vi "Setup.vi"(8 "Error In":errorcluster, 10 "Data":refnum<class "Datum.lvclass">, 11 "Value":string) -> (0 "Error Out":errorcluster, 2 "Abstract Syntax Tree":refnum<class "Root.lvclass">, 3 "Renderer":refnum<class "Renderer.lvclass">)   [LabVIEW 2018, in "Tests.lvlib" / "Render.lvlib"]
uses:
  Render.lvlib
  src/Toolkit/Low-Level/Nodes/Root/Root.lvclass
  src/Toolkit/Low-Level/Renderer/Renderer.lvclass
  src/Toolkit/Data/Datum/Datum.lvclass
  src/Toolkit/Low-Level/Writers/String/String.lvclass
  D:/Users/cfield/Code/Field R&D Services/Labstache/src/Toolkit/Low-Level/Writers/Writer/Writer.lvclass
  src/Toolkit/Low-Level/Readers/String/String.lvclass
  D:/Users/cfield/Code/Field R&D Services/Labstache/src/Toolkit/Low-Level/Readers/Reader/Reader.lvclass
  src/Toolkit/Low-Level/Lexer/Lexer.lvclass
  src/Toolkit/Low-Level/Parser/Parser.lvclass
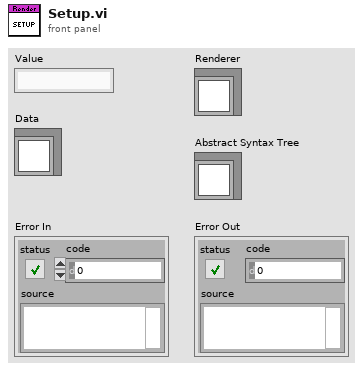
[diagram p1: front panel]
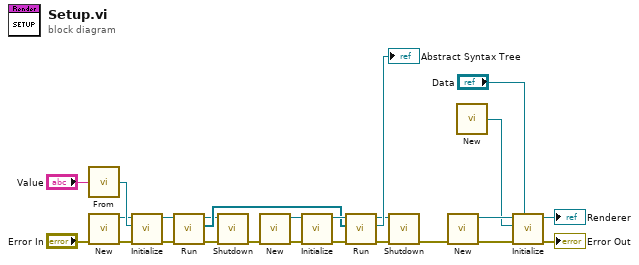
[diagram p0: block diagram]
diagram:
  n1 = call "From.vi"("Value"="Value") -> ("String"=w3:refnum<class "String.lvclass">)
  n2 = call "New.vi"("Error In"="Error In") -> ("Error Out"=w1:errorcluster, "Lexer"=w2:refnum<class "Lexer.lvclass">)  [unwired: 9 in]
  n3 = call-dynamic "Initialize.vi"("Error In"=w1, "Reader"=w3, "Lexer In"=w2) -> ("Error Out"=w11:errorcluster, "Lexer Out"=w10:refnum<class "Lexer.lvclass">)  [unwired: 7 in]
  n4 = call-dynamic "Run.vi"("Error In"=w11, "Lexer In"=w10) -> ("Error Out"=w12:errorcluster, "Tokens"=w14:refnum<class "Token.lvclass">[], "Lexer Out"=w13:refnum<class "Lexer.lvclass">)  [unwired: 7 in]
  n5 = call-dynamic "Shutdown.vi"("Error In"=w12, "Lexer In"=w13) -> ("Error Out"=w19:errorcluster)  [unwired: 7 in, 2 out]
  n6 = call "New.vi"("Error In"=w19) -> ("Error Out"=w20:errorcluster, "Parser"=w21:refnum<class "Parser.lvclass">)  [unwired: 9 in]
  n7 = call-dynamic "Initialize.vi"("Error In"=w20, "Parser In"=w21) -> ("Error Out"=w16:errorcluster, "Parser Out"=w15:refnum<class "Parser.lvclass">)  [unwired: 8 in]
  n8 = call-dynamic "Run.vi"("Error In"=w16, "Tokens"=w14, "Parser In"=w15) -> ("Error Out"=w17:errorcluster, "Abstract Syntax Tree"=→"Abstract Syntax Tree":refnum<class "Root.lvclass">, "Parser Out"=w18:refnum<class "Parser.lvclass">)  [unwired: 6 in]
  n9 = call-dynamic "Shutdown.vi"("Error In"=w17, "Parser In"=w18) -> ("Error Out"=w22:errorcluster)  [unwired: 8 in, 1 out]
  n10 = call "New.vi"("Error In"=w22) -> ("Error Out"=w5:errorcluster, "Renderer"=w6:refnum<class "Renderer.lvclass">)  [unwired: 9 in]
  n11 = call "New.vi"() -> ("String Writer"=w4:refnum<class "String.lvclass">)  [unwired: 1 in]
  n12 = call-dynamic "Initialize.vi"("Data"="Data", "Error In"=w5, "Writer"=w4, "Renderer In"=w6) -> ("Error Out"=→"Error Out":errorcluster, "Renderer Out"=→"Renderer":refnum<class "Renderer.lvclass">)  [unwired: 6 in]
